vi "Dist to Stop at 0.4.vi"(10 "Speed":dbl format="%#_13g") -> (2 "Distance":i32)   [LabVIEW 2017]
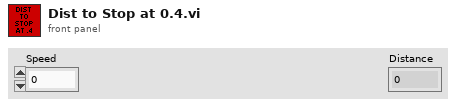
[diagram p1: front panel]
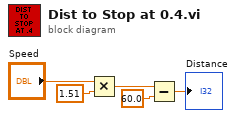
[diagram p0: block diagram]
diagram:
  n1 = Multiply(x="Speed", y=1.51) -> (x*y=w3:dbl)
  n2 = Subtract(x=w3, y=60.0) -> (x-y=→"Distance":dbl)
